vi "Sets_Union(U64).vi"(8 "error in (no error)":errorcluster caption="错误输入（无错误）", 10 "输入数组B":u64[](array[numeric]), 11 "输入数组A":u64[](array[numeric])) -> (0 "error out":errorcluster caption="错误输出", 3 "输出数组C":u64[](array[numeric]))   [LabVIEW 2011]
uses:
  Sets_Unique(U64).vi
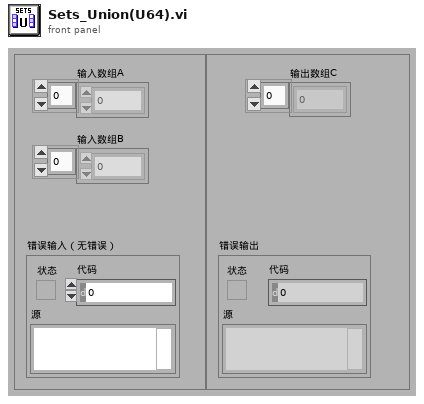
[diagram p1: front panel]
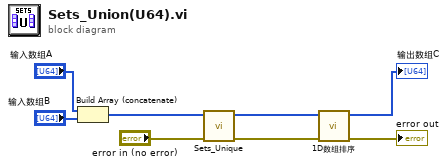
[diagram p0: block diagram]
diagram:
  n1 = Build Array (concatenate)("输入数组A", "输入数组B") -> (w4:u64[])
  n2 = call-poly "Sets_Unique.vi"("error in (no error)"="error in (no error)", "输入数组"=w4) -> ("error out"=w2:errorcluster, "输出数组"=w3:u64[])  [unwired: 7 in, 1 out]
  n3 = call-poly "1D数组排序.vi"("error in (no error)"=w2, "输入数组"=w3) -> ("error out"=→"error out":errorcluster, "排序后数组"=→"输出数组C":u64[])  [unwired: 7 in, 1 out]
